vi "module-05-on-off-delay-one-shot.vi"() -> ()   [LabVIEW 2019]
uses:
  <vilib>/Rock Robotics/WPI/ThirdParty/JAS_Junk/TrajLib/Timer_New.vi
  <vilib>/Rock Robotics/WPI/ThirdParty/JAS_Junk/TrajLib/Timer_Start.vi
  <vilib>/Rock Robotics/WPI/ThirdParty/JAS_Junk/TrajLib/Timer_HasPeriodPassedOnce.vi
  samples-common-library/Ctrl_Training_Library_Protected/CtrlTrainingLibary_Protected.lvlib
panel:
  in  "Tab Control":enum32{"Control Panel", "Logic"}(tab)
  in  "Input":bool
  out "On Delay\nOutput":bool
  in  "On Delay\nTime":dbl=10.0
  out "On Delay\nRemaining":dbl
  in  "Off Delay\nTime":dbl=3.0
  out "Off Delay\nOutput":bool
  out "Off Delay\nRemaining":dbl
  out "One Shot\nOutput":bool
  out "One Shot\nRemaining":dbl
  in  "One Shot\nTime":dbl=5.0
  out "Digital State Chart":cluster{dbl, dbl, dbl, dbl, dbl, dbl}(graph)
  # "ON DELAY, OFF DELAY,\nONE SHOT  TEST"
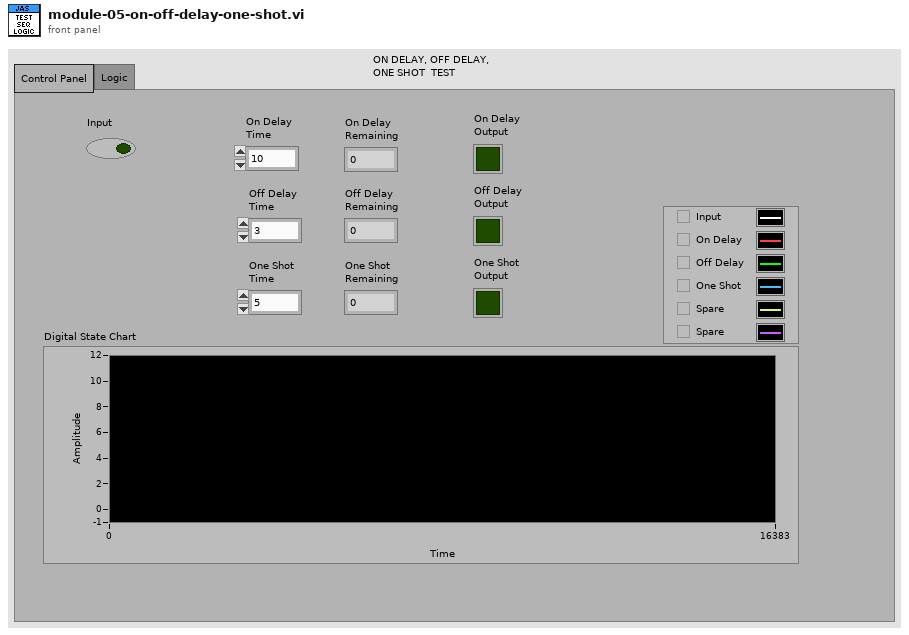
[diagram p1: front panel]
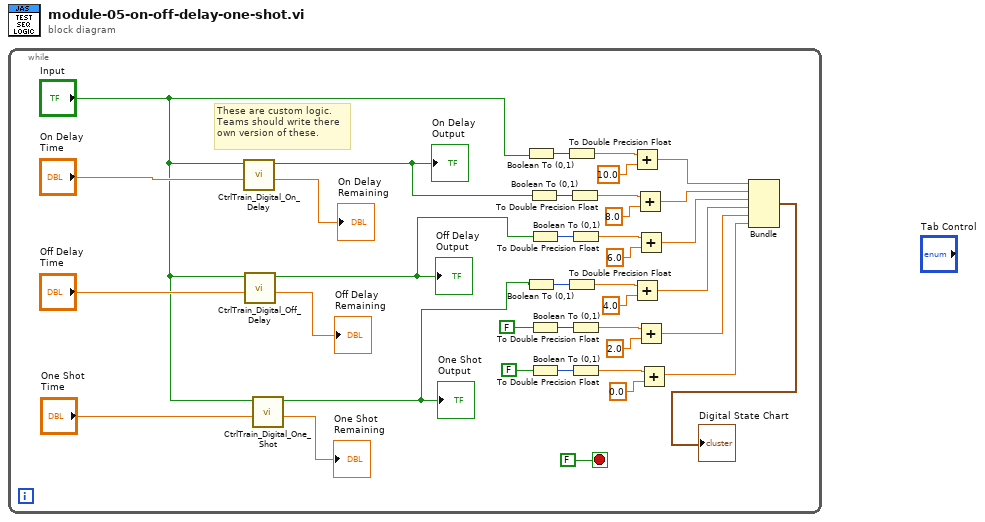
[diagram p0: block diagram]
diagram:
  n1 = while {
    stop <- FALSE stop-if-true
    # "These are custom logic.\nTeams should write there\nown version of these."
    n2 = call "CtrlTrain_Digital_On_Delay.vi"("Delay"="On Delay\nTime", "Input"="Input") -> ("Remain"=→"On Delay\nRemaining":dbl, "Output"=w4:bool)  [unwired: 8 in]
    "On Delay\nOutput" <- w4
    n3 = call "CtrlTrain_Digital_Off_Delay.vi"("Delay"="Off Delay\nTime", "Input"="Input") -> ("Remain"=→"Off Delay\nRemaining":dbl, "Output"=w3:bool)  [unwired: 8 in]
    "Off Delay\nOutput" <- w3
    n4 = call "CtrlTrain_Digital_One_Shot.vi"("OneShot"="One Shot\nTime", "Input"="Input") -> ("Remain"=→"One Shot\nRemaining":dbl, "Output"=w2:bool)  [unwired: 8 in]
    "One Shot\nOutput" <- w2
    n5 = Boolean To (0,1)(Boolean="Input") -> (0, 1=w14:i16)
    n6 = Boolean To (0,1)(Boolean=w2) -> (0, 1=w15:i16)
    n7 = Boolean To (0,1)(Boolean=w4) -> (0, 1=w17:i16)
    n8 = Boolean To (0,1)(Boolean=w3) -> (0, 1=w19:i16)
    n9 = Boolean To (0,1)(Boolean=FALSE) -> (0, 1=w21:i16)
    n10 = Boolean To (0,1)(Boolean=FALSE) -> (0, 1=w23:i16)
    n11 = To Double Precision Float(number=w14) -> (double precision float=w30:dbl)
    n12 = To Double Precision Float(number=w15) -> (double precision float=w16:dbl)
    n13 = To Double Precision Float(number=w17) -> (double precision float=w18:dbl)
    n14 = To Double Precision Float(number=w19) -> (double precision float=w20:dbl)
    n15 = To Double Precision Float(number=w21) -> (double precision float=w22:dbl)
    n16 = To Double Precision Float(number=w23) -> (double precision float=w24:dbl)
    n17 = Add(x=w30, y=10.0) -> (x+y=w31:dbl)
    n18 = Add(x=w16, y=4.0) -> (x+y=w29:dbl)
    n19 = Add(x=w18, y=8.0) -> (x+y=w27:dbl)
    n20 = Add(x=w20, y=6.0) -> (x+y=w28:dbl)
    n21 = Add(x=w22, y=2.0) -> (x+y=w25:dbl)
    n22 = Add(x=w24, y=0.0) -> (x+y=w26:dbl)
    n23 = Bundle(w31, w27, w28, w29, w25, w26) -> (→"Digital State Chart":cluster{dbl, dbl, dbl, dbl, dbl, dbl})  [unwired: 1 in]
  }
